vi "Rawdata_Imagedata_Generator.vi"() -> ()   [LabVIEW 2020]
uses:
  ctl/Image_Configuration.ctl
  ctl/Image_RAW_Bayer_Pattern.ctl
panel:
  out "Image":T1(plugin-control)
  in  "stop":bool
  out "Progress":dbl(slide) scale=0.0..100.0
  out "error out":errorcluster
  in  "Output File Path":path
  in  "Num of Frames to generate":u32=30
  in  "Pattern Color List":u32[](array[colorbox])=[0, 16777215, 16711680, 255, 65280, 16711935, 32768, 8388736, 12632256, 14423100, 128, 16766720, 8388608, 65535, 16761035, 8421376, 16742144, 8421504, 16729344, 25600, 16777200, 4915330, 15787660, 49151, 6908265, 9498256, 16716947, 4286975, 10824234, 35723]
  in  "Bayer Pattern":T2=enum."RGGB (GRBG)"
  in  "Image Data Type":u8=44 format="%x"
  in  "Image Configuration":T3={"Width"=1920, "Height"=1536}
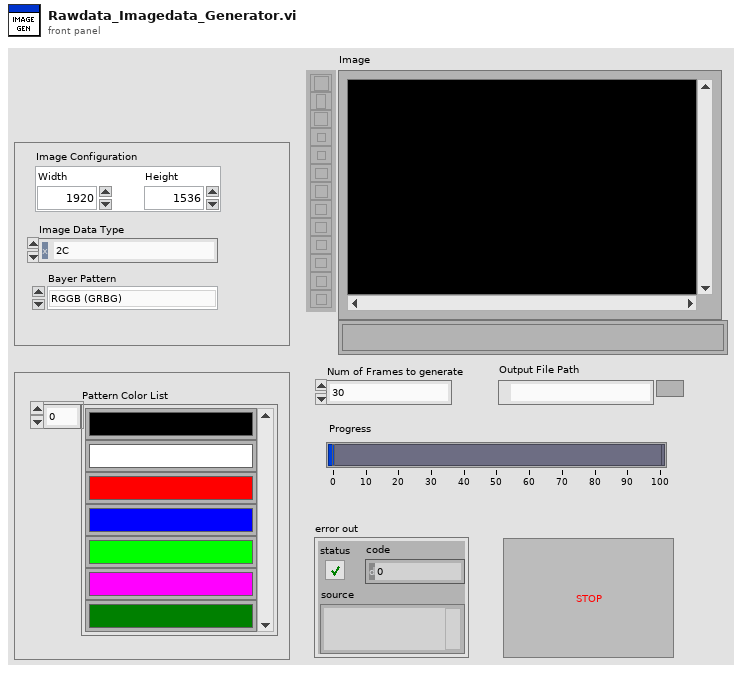
[diagram p1: front panel]
types:
  T1 = typedef "IMAQ Image.ctl" = refnum<image>
  T2 = typedef "Image_RAW_Bayer_Pattern.ctl" = enum16{"GBRG (BGGR)", "GRBG (RGGB)", "BGGR (GBRG)", "RGGB (GRBG)", "CRBC (RCCB)"}
  T3 = typedef "Image_Configuration.ctl" = cluster{"Width":i32, "Height":i32}
  T4 = enum16{"open", "replace", "create", "open or create", "replace or create", "replace or create with confirmation"}
  T5 = enum16{"big-endian, network order", "native, host order", "little-endian"}
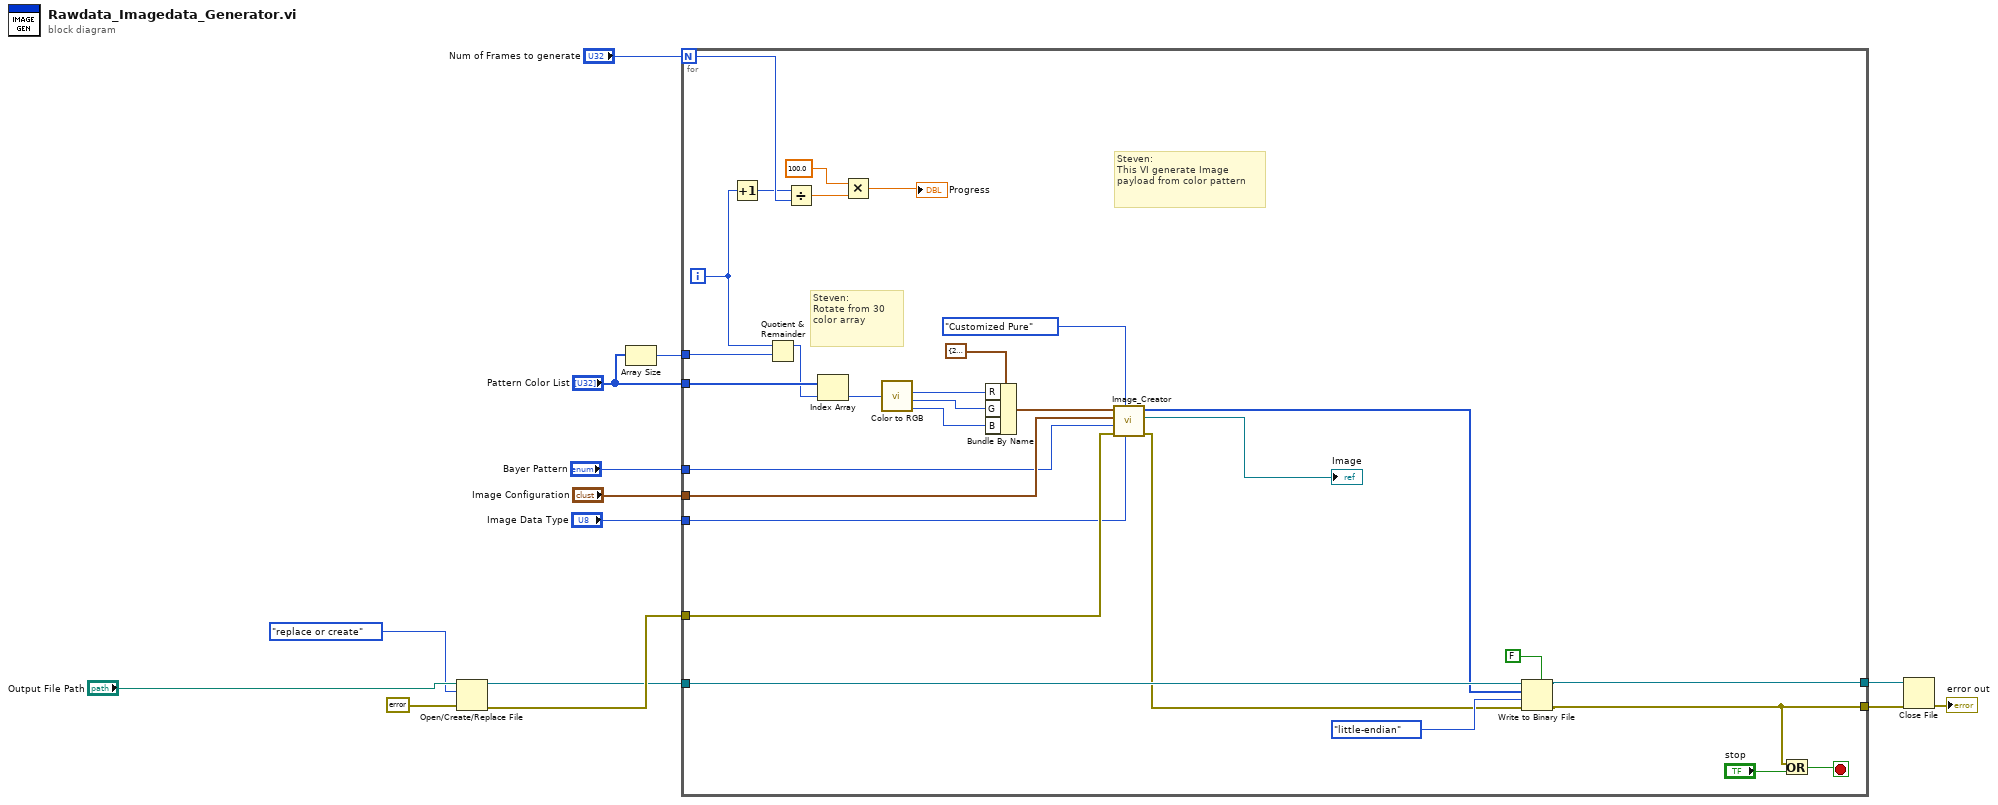
[diagram p0: block diagram]
diagram:
  n1 = Open/Create/Replace File(file path (use dialog)="Output File Path", error in=errorcluster {"status"=FALSE, "code"=0, "source"=""} ("error in (no error)"), operation (0:open)=T4."replace or create") -> (refnum out=w4:refnum<file>, error out=w5:errorcluster)  [unwired: 3 in, 1 out]
  n2 = Array Size(array="Pattern Color List") -> (size(s)=w10:i32)
  n3 = for {
    N: "Num of Frames to generate" -> [w27]
    tunnel: "Image Configuration" -> [w34]
    tunnel: "Pattern Color List" -> [w43]
    tunnel: w10 -> [w44]
    tunnel: "Bayer Pattern" -> [w33]
    tunnel: "Image Data Type" -> [w20]
    tunnel: w5 -> [w32]
    tunnel: w4 -> [w31]
    tunnel: [w19] -> w3
    tunnel: [w18] -> w2
    i -> [w28]
    stop <- w22 stop-if-true
    # "Steven:\nRotate from 30 color array"
    # "Steven:\nThis VI generate Image payload from color pattern"
    n4 = Increment(x=w28) -> (x+1=w21:i32)
    n5 = Quotient & Remainder(x=w28, y=w44) -> (x-y*floor(x/y)=w42:i32)  [unwired: 1 out]
    n6 = Divide(x=w21, y=w27) -> (x/y=w26:dbl)
    n7 = Index Array(array=w43, index=w42) -> (element=w41:u32)
    n8 = Multiply(x=100.0, y=w26) -> (x*y=→"Progress":dbl)
    n9 = call <vilib>:"Color to RGB.vi"("Color"=w41) -> ("R"=w39:u8, "G"=w38:u8, "B"=w37:u8)  [unwired: 1 out]
    n10 = Bundle By Name(cluster=cluster{"R":u8, "G":u8, "B":u8} {"R"=255, "G"=255, "B"=255} ("Pure Color Pattern Parameters"), "R"=w39, "G"=w38, "B"=w37) -> (w36:cluster{"R":u8, "G":u8, "B":u8})
    n11 = call "Image_Creator.vi"("Image Data Type"=w20, "Pattern"=enum16{"24 Color Checker", "Customized Pure"}."Customized Pure", "error in (no error)"=w32, "Bayer Pattern"=w33, "Image Configuration"=w34, "Pure Color Pattern Parameters"=w36) -> ("error out"=w15:errorcluster, "Image"=→"Image":T1, "Image Data Payload (U8)"=w16:u8[])  [unwired: 2 in, 1 out]
    n12 = Write to Binary File(file (use dialog)=w31, data=w16, error in=w15, 5:FALSE ("prepend array or string size? (T)"), 9:T5."little-endian" ("byte order (0:big-endian, network order)")) -> (refnum out=w19:refnum<file>, error out=w18:errorcluster)  [unwired: 1 in, 1 out]
    n13 = Or(x=w18, y="stop") -> (x .or. y?=w22:bool)
  }
  n14 = Close File(refnum=w3, error in=w2) -> (error out=→"error out":errorcluster)  [unwired: 1 out]
